vi "RemovePeaks2.vi"(11 "wfm in":waveform(dbl)) -> (2 "original + denoised":waveform(dbl)[](graph), 3 "denoised wfm":waveform(dbl)(graph))   [LabVIEW 2025]
uses:
  <vilib>/gmath/statdist.llb/st_Percentiles (scalar).vi
  <vilib>/gmath/NI_Gmath.lvlib
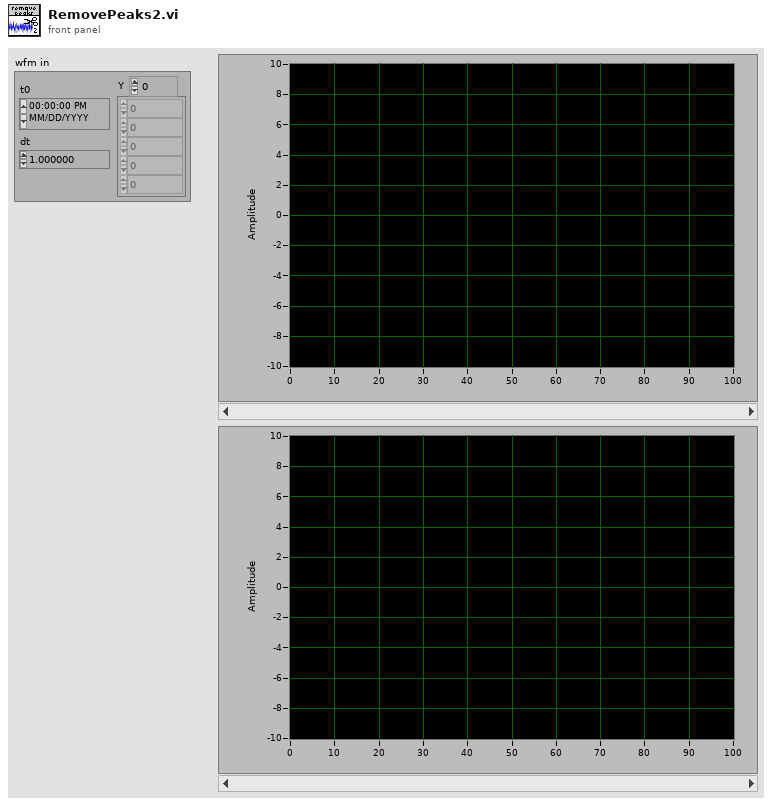
[diagram p1: front panel]
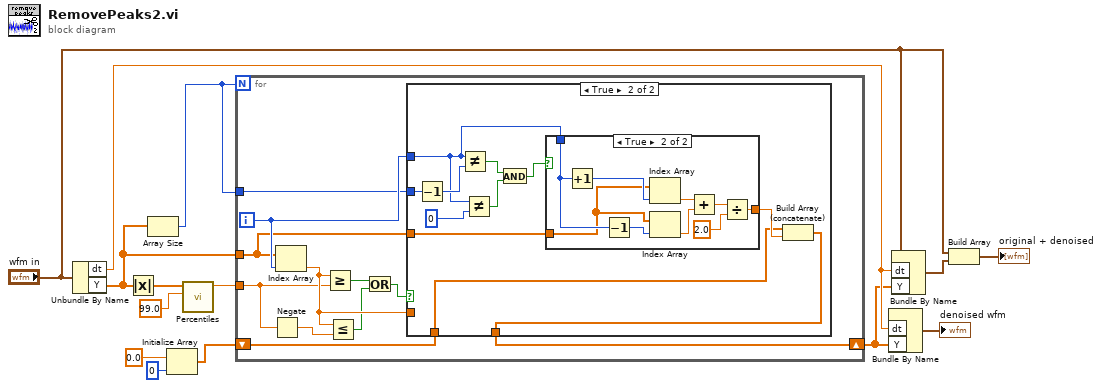
[diagram p0: block diagram]
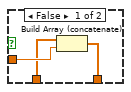
[diagram p2: hidden frame]
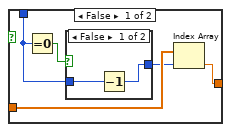
[diagram p3: hidden frame]
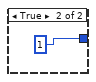
[diagram p4: hidden frame]
diagram:
  n1 = Unbundle By Name("wfm in") -> ("dt"=w9:dbl, "Y"=w12:dbl[])
  n2 = Absolute Value(x=w12) -> (abs(x)=w13:dbl[])
  n3 = Array Size(array=w12) -> (size(s)=w1:i32)
  n4 = Initialize Array(0.0 ("element"), 0 ("dimension size")) -> (w2:dbl[])
  n5 = call-poly <vilib>:"Percentiles.vi"("p"=99.0, "x array"=w13) -> ("percentile"=w11:dbl)  [unwired: 8 in, 1 out]
  n6 = for {
    N: w1 -> [_]
    tunnel: w12 -> [w15]
    tunnel: w11 -> [w21]
    shift-right: [w25] -> w8
    shift-left: w2 -> [w24]
    tunnel: w1 -> [w16]
    i -> [w17]
    n7 = Negate(x=w21) -> (-x=w22:dbl)
    n8 = Index Array(array=w15, index=w17) -> (element=w23:dbl)
    n9 = Greater Or Equal?(x=w23, y=w21) -> (x >= y?=w20:bool)
    n10 = Less Or Equal?(x=w23, y=w22) -> (x <= y?=w19:bool)
    n11 = Or(x=w20, y=w19) -> (x .or. y?=w18:bool)
    n12 = case shown="True" w18 {
      tunnel: w23 -> [w27 _]
      tunnel: [w28 w30] -> w25
      tunnel: w24 -> [w26 w31]
      tunnel: w17 -> [_ w29]
      tunnel: w16 -> [_ w34]
      tunnel: w15 -> [_ w33]
      frame False {
        n13 = Build Array (concatenate)(w26, w27) -> (w28:dbl[])
      }
      frame True {
        n14 = Decrement(x=w34) -> (x-1=w39:i32)
        n15 = Not Equal?(x=w29, y=w39) -> (x != y?=w37:bool)
        n16 = Not Equal?(x=w29, y=0) -> (x != y?=w36:bool)
        n17 = And(x=w37, y=w36) -> (x .and. y?=w35:bool)
        n18 = case shown="True" w35 {
          tunnel: w33 -> [w42 w53]
          tunnel: w29 -> [w40 w54]
          tunnel: [w43 w48] -> w32
          frame False {
            n19 = Equal To 0?(x=w40) -> (x = 0?=w44:bool)
            n20 = case shown="False" w44 {
              tunnel: [w45 1] -> w41
              tunnel: w40 -> [w46 _]
              frame False {
                n21 = Decrement(x=w46) -> (x-1=w45:i32)
              }
              frame True {
              }
            }
            n22 = Index Array(array=w42, index=w41) -> (element=w43:dbl)
          }
          frame True {
            n23 = Increment(x=w54) -> (x+1=w56:i32)
            n24 = Decrement(x=w54) -> (x-1=w55:i32)
            n25 = Index Array(array=w53, index=w56) -> (element=w52:dbl)
            n26 = Index Array(array=w53, index=w55) -> (element=w51:dbl)
            n27 = Add(x=w52, y=w51) -> (x+y=w50:dbl)
            n28 = Divide(x=w50, y=2.0) -> (x/y=w48:dbl)
          }
        }
        n29 = Build Array (concatenate)(w31, w32) -> (w30:dbl[])
      }
    }
  }
  n30 = Bundle By Name("dt"=w9, "Y"=w8) -> (→"denoised wfm":waveform(dbl))  [unwired: 1 in]
  n31 = Bundle By Name(cluster="wfm in", "dt"=w9, "Y"=w8) -> (w6:waveform(dbl))
  n32 = Build Array("wfm in", w6) -> (→"original + denoised":waveform(dbl)[])
